vi "Shell and Tube Heat Exchanger 3.vi"() -> ()   [LabVIEW 2017]
uses:
  <vilib>/addons/control/pid/pid.llb/PID Control Input Filter (DBL).vi
  <vilib>/addons/control/pid/pid.llb/PID Advanced (DBL).vi
  <vilib>/addons/control/pid/NI_PID_pid.lvlib
panel:
  in  "stop":bool
  in  "Recording Increment (sec)":dbl=0.3 min=0.1 max=100.0 step=0.1 format="%#_13g"
  in  "error in":errorcluster
  out "Last Time Write":dbl
  in  "Replace File":bool
  out "Makeup Flowrate":dbl caption="L/min"
  out "Makeup Temperature":dbl caption="C"
  in  "Pump Switch":bool
  out "Water Outlet Temperature":dbl=22.816489944987293 format="%.1f"
  in  "Flowrate Setpoint (GPM)":dbl=40.0 min=0.0 max=50.0 format="%.2f"
  out "Water Flowrate":dbl=-0.0005338564515105265 format="%.2f"
  out "Flow Control Valve":dbl(slide)=100.0 scale=0.0..100.0
  in  "Manual Control Override (Flow)":bool=TRUE
  in  "Set Manual Valve Position (Flow)":dbl(slide)=100.0 scale=0.0..100.0
  in  "Level Setpoint (ft)":dbl=1.5 min=0.0 max=2.0 format="%.2f"
  out "Liquid Level in Tank":dbl=-0.5117058749718749 format="%.2f"
  out "Level Control Valve":dbl(slide)=0.045055175643920364 scale=0.0..100.0
  in  "Manual Control Override (Level)":bool=TRUE
  in  "Set Manual Valve Position (Level)":dbl(slide) scale=0.0..100.0
  in  "Kc (Flow)":dbl=0.74
  in  "Ti (Flow)":dbl=0.036 caption="(min)"
  in  "Td (Flow)":dbl caption="(min)"
  in  "Kc (Level)":dbl=-75.0
  in  "Ti (Level)":dbl=0.005 caption="(min)"
  in  "Td (Level)":dbl caption="(min)"
  out "House Steam Pressure":dbl=-37.74410859375 caption="psig" format="%#.6g"
  out "Tube-Side Pressure Drop":dbl=-3.6907662628125 caption="psig"
  in  "Main Power":bool
  out "Water Feed Temperature":dbl=19.10777415276108 caption="C"
  in  "Steam Pressure Setpoint (psig)":dbl=10.0 min=0.0 max=45.0 format="%.2f"
  out "Steam Pressure":dbl=-38.330115825 caption="psig" format="%.2f"
  out "Steam Valve":dbl(slide) scale=0.0..100.0
  in  "Manual Control Override (Steam Pressure)":bool
  in  "Set Manual Valve Position (Steam Pressure)":dbl(slide) scale=0.0..100.0
  in  "Kc (Steam)":dbl=0.5
  in  "Ti (Steam)":dbl=0.05 caption="(min)"
  in  "Td (Steam)":dbl caption="(min)"
  in  "Enable 5":bool
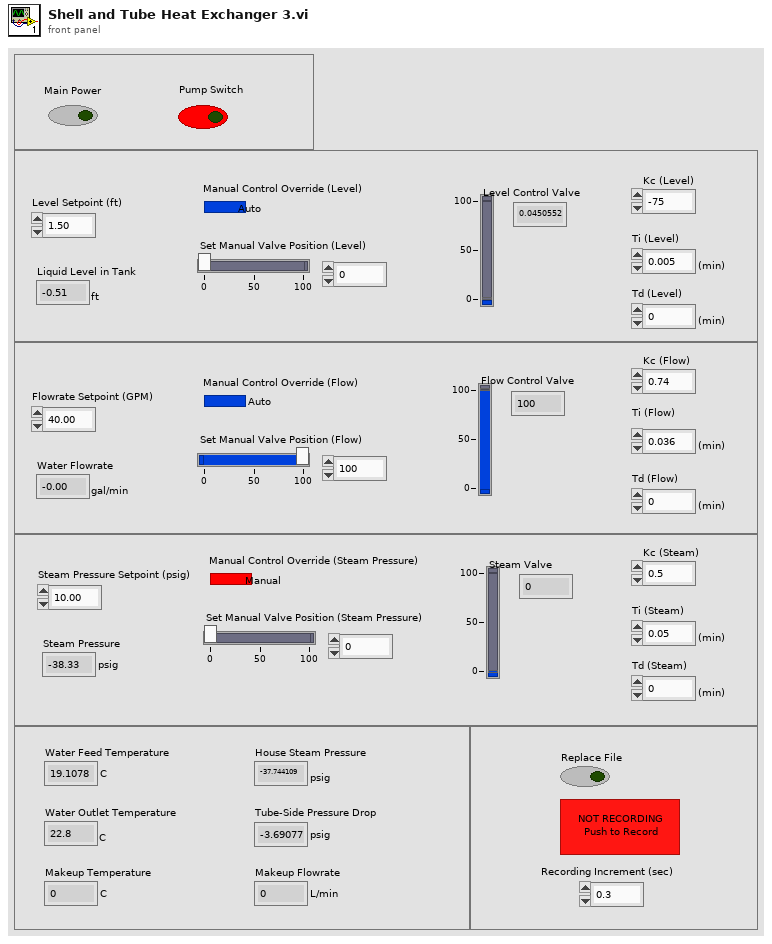
[diagram p1: front panel]
types:
  T1 = enum16{"open", "replace", "create", "open or create", "replace or create", "replace or create with confirmation"}
  T2 = cluster{"Kc (Flow)":dbl, "Ti (Flow)":dbl, "Td (Flow)":dbl}
  T3 = cluster{"Kc (Steam)":dbl, "Ti (Steam)":dbl, "Td (Steam)":dbl}
  T4 = cluster{"Kc (Level)":dbl, "Ti (Level)":dbl, "Td (Level)":dbl}
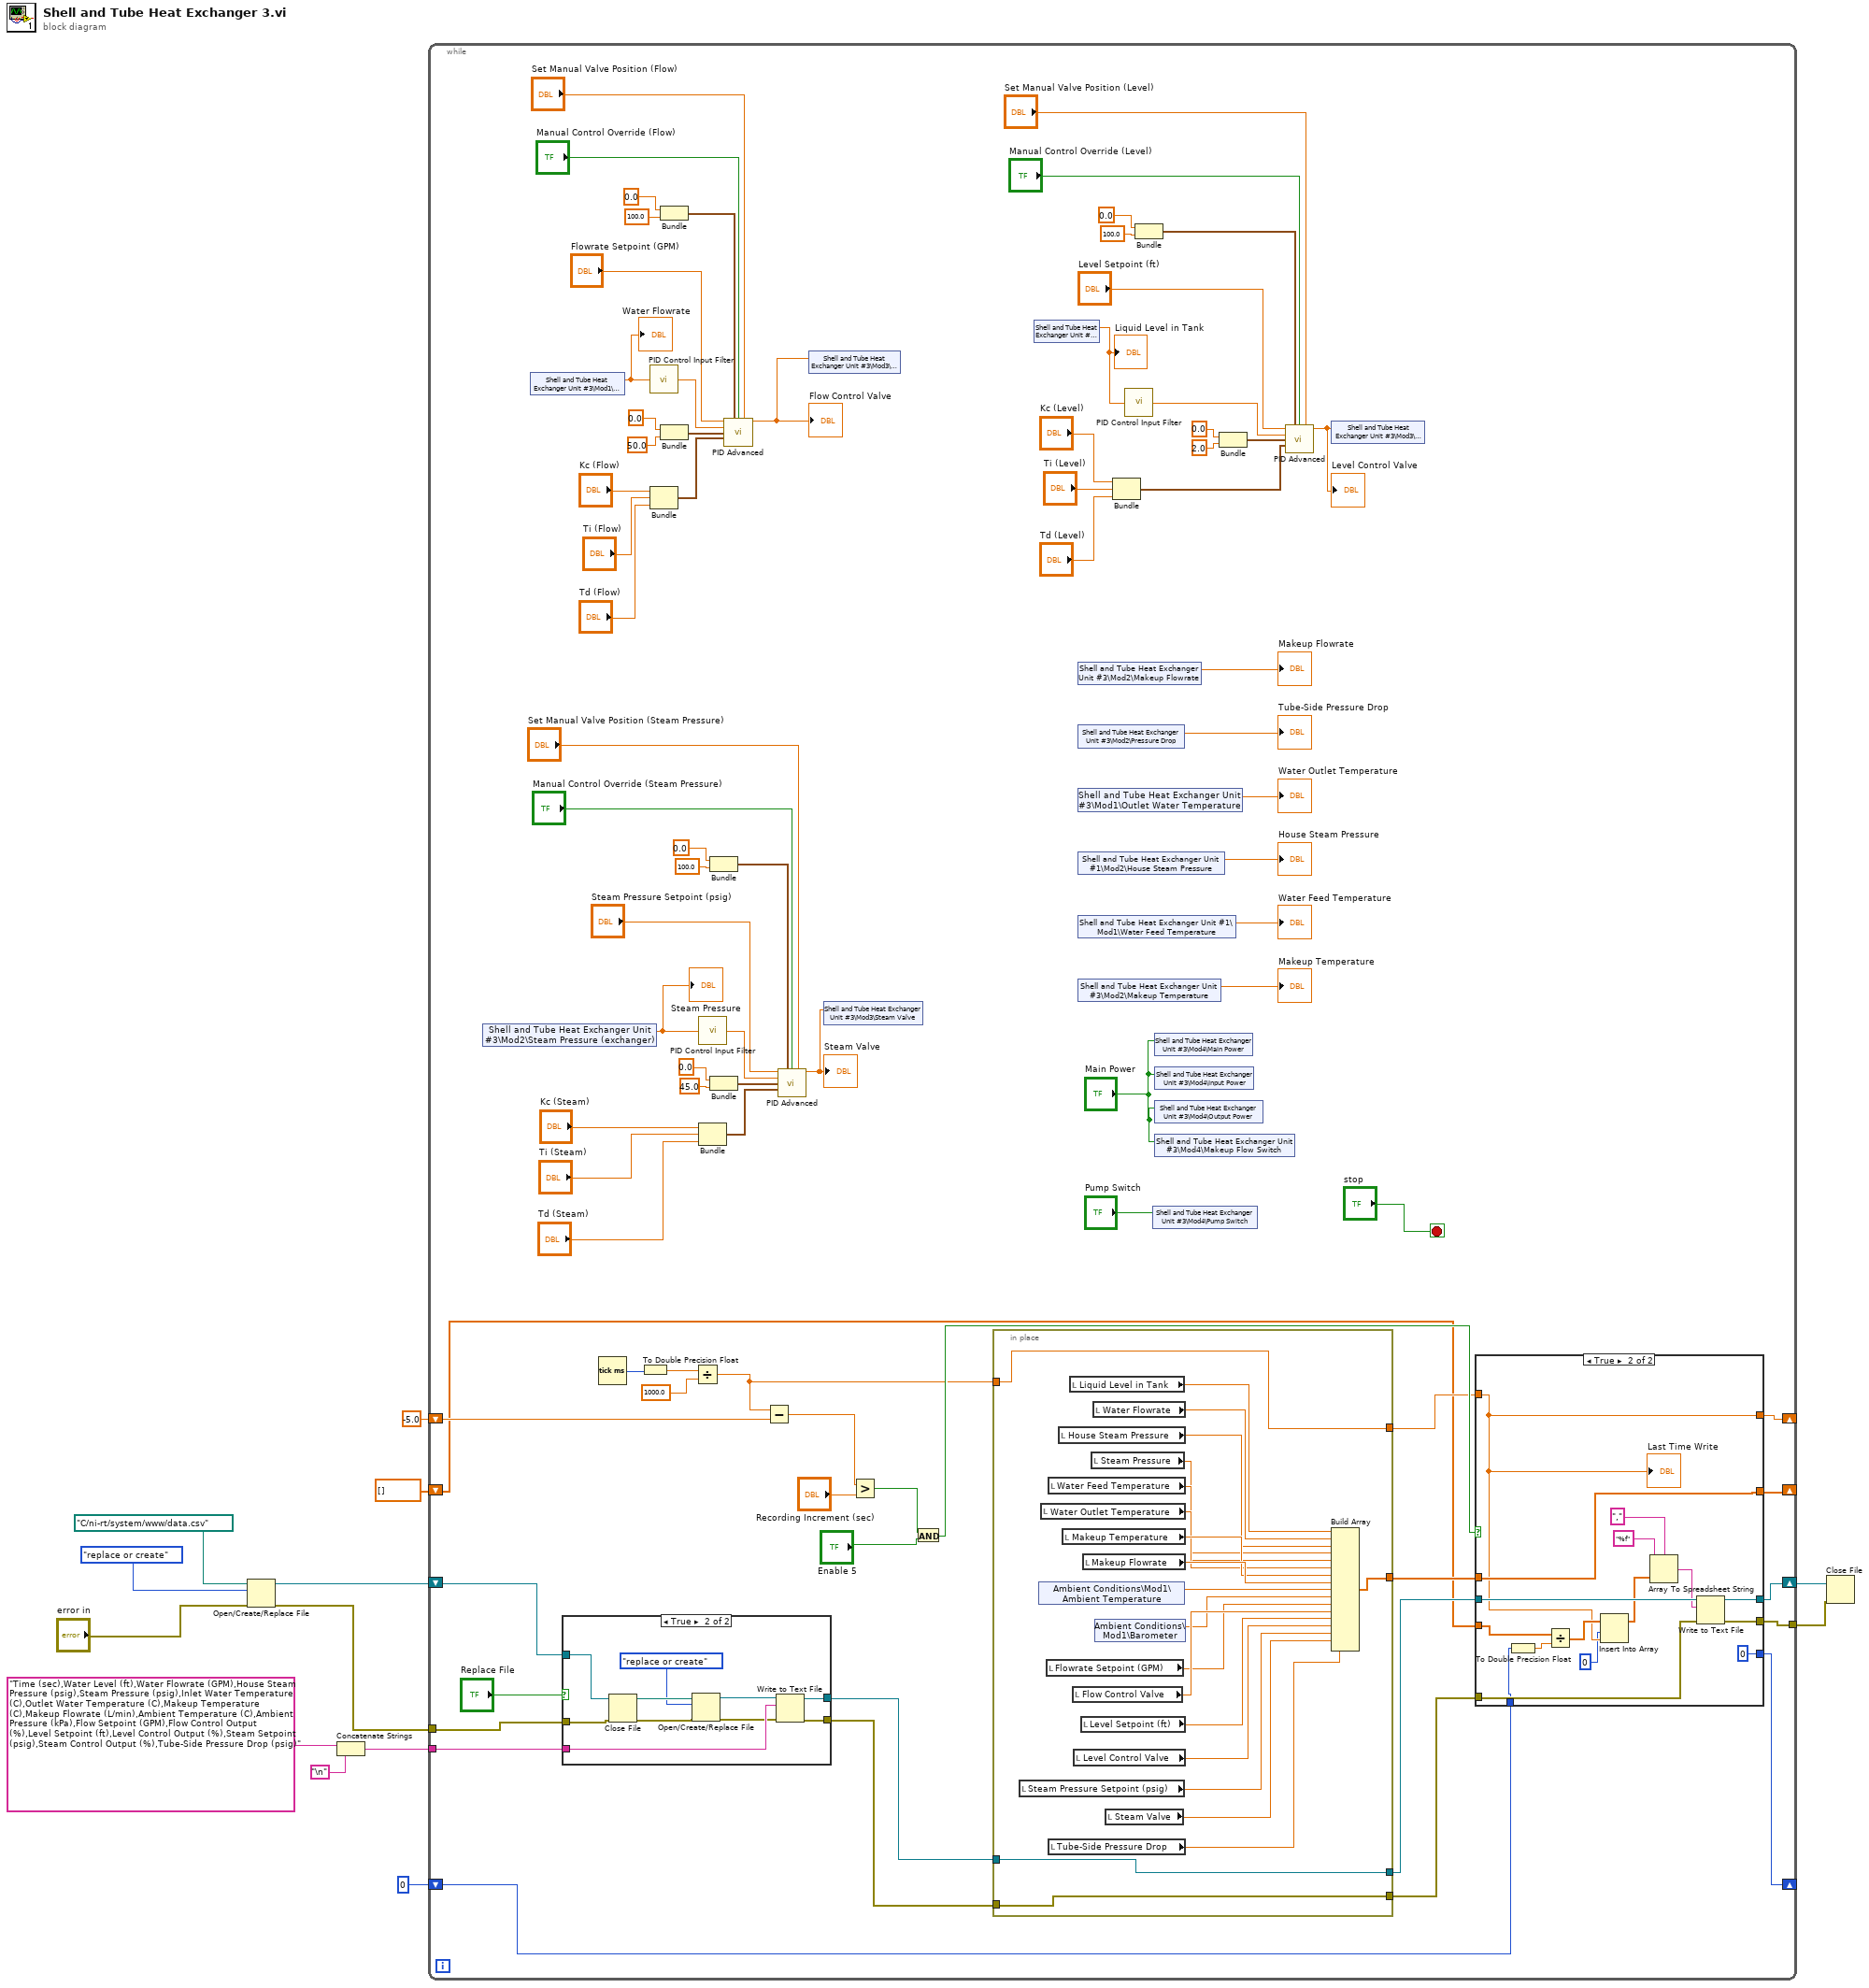
[diagram p0: block diagram]
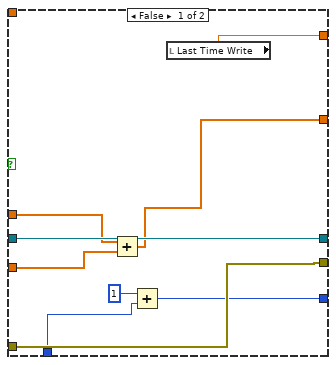
[diagram p2: hidden frame]
diagram:
  n1 = Open/Create/Replace File(file path (use dialog)=path "C:/ni-rt/system/www/data.csv" ("Filename"), error in="error in", operation (0:open)=T1."replace or create") -> (refnum out=w10:refnum<file>, error out=w5:errorcluster)  [unwired: 3 in, 1 out]
  n2 = Concatenate Strings("Time (sec),Water Level (ft),Water Flowrate (GPM),House Steam Pressure (psig),Steam Pressure (psig),Inlet Water Temperature (C),Outlet Water Temperature (C),Makeup Temperature (C),Makeup Flowrate (L/min),Ambient Temperature (C),Ambient Pressure (kPa),Flow Setpoint (GPM),Flow Control Output (%),Level Setpoint (ft),Level Control Output (%),Steam Setpoint (psig),Steam Control Output (%),Tube-Side Pressure Drop (psig)", "\n") -> (w8:string)
  n3 = while {
    tunnel: w8 -> [w41]
    shift-right: [w31] -> _
    shift-left: -5.0 ("Last Time Write") -> [w34]
    shift-right: [w29] -> w7
    shift-left: w10 -> [w40]
    tunnel: w5 -> [w28]
    tunnel: [w27] -> w4
    shift-right: [w17] -> _
    shift-left: dbl[] [] -> [w16]
    shift-right: [w14] -> _
    shift-left: 0 -> [w15]
    stop <- "stop" stop-if-true
    n4 = shared-variable "Shell and Tube Heat Exchanger Unit #3\\Mod2\\Steam Pressure (exchanger)"() -> (w52:dbl)  [unwired: 1 in, 1 out]
    "Steam Pressure" <- w52
    n5 = shared-variable "Shell and Tube Heat Exchanger Unit #3\\Mod1\\Water Flow"() -> (w54:dbl)  [unwired: 1 in, 1 out]
    "Water Flowrate" <- w54
    n6 = case shown="True" "Replace File" {
      tunnel: w41 -> [_ w153]
      tunnel: w40 -> [w145 w151]
      tunnel: [w145 w150] -> w21
      tunnel: w28 -> [w144 w149]
      tunnel: [w144 w146] -> w23
      frame False {
      }
      frame True {
        n7 = Close File(refnum=w151, error in=w149) -> (path=w154:path, error out=w148:errorcluster)
        n8 = Open/Create/Replace File(file path (use dialog)=w154, error in=w148, operation (0:open)=T1."replace or create") -> (refnum out=w155:refnum<file>, error out=w147:errorcluster)  [unwired: 3 in, 1 out]
        n9 = Write to Text File(file (use dialog)=w155, text=w153, error in=w147) -> (refnum out=w150:refnum<file>, error out=w146:errorcluster)  [unwired: 1 in, 1 out]
      }
    }
    n10 = Tick Count (ms)() -> (millisecond timer value=w33:u32)
    n11 = To Double Precision Float(number=w33) -> (double precision float=w32:dbl)
    n12 = call-poly <vilib>:"PID Control Input Filter.vi"("input"=w54) -> ("output"=w53:dbl)  [unwired: 4 in]
    n13 = Bundle("Kc (Flow)"="Kc (Flow)", "Ti (Flow)"="Ti (Flow)", "Td (Flow)"="Td (Flow)") -> (w93:T2)  [unwired: 1 in]
    n14 = Bundle(0.0, 100.0) -> (w78:cluster{dbl, dbl})  [unwired: 1 in]
    n15 = Bundle(0.0, 50.0) -> (w75:cluster{dbl, dbl})  [unwired: 1 in]
    n16 = Divide(x=w32, y=1000.0) -> (x/y=w19:dbl)
    n17 = call-poly <vilib>:"PID Control Input Filter.vi"("input"=w52) -> ("output"=w51:dbl)  [unwired: 4 in]
    n18 = Bundle("Kc (Steam)"="Kc (Steam)", "Ti (Steam)"="Ti (Steam)", "Td (Steam)"="Td (Steam)") -> (w67:T3)  [unwired: 1 in]
    n19 = Bundle(0.0, 100.0) -> (w62:cluster{dbl, dbl})  [unwired: 1 in]
    n20 = Bundle(0.0, 45.0) -> (w59:cluster{dbl, dbl})  [unwired: 1 in]
    n21 = call-poly <vilib>:"PID Advanced.vi"("setpoint"="Flowrate Setpoint (GPM)", "output range"=w78, "auto? (T)"="Manual Control Override (Flow)", "manual control"="Set Manual Valve Position (Flow)", "process variable"=w53, "setpoint range"=w75, "PID gains"=w93) -> ("output"=w49:dbl)  [unwired: 7 in, 1 out]
    "Flow Control Valve" <- w49
    n22 = Subtract(x=w19, y=w34) -> (x-y=w35:dbl)
    n23 = call-poly <vilib>:"PID Advanced.vi"("setpoint"="Steam Pressure Setpoint (psig)", "output range"=w62, "auto? (T)"="Manual Control Override (Steam Pressure)", "manual control"="Set Manual Valve Position (Steam Pressure)", "process variable"=w51, "setpoint range"=w59, "PID gains"=w67) -> ("output"=w46:dbl)  [unwired: 7 in, 1 out]
    "Steam Valve" <- w46
    n24 = shared-variable "Shell and Tube Heat Exchanger Unit #3\\Mod3\\Flow Valve"(w49) -> ()  [unwired: 1 in, 1 out]
    n25 = shared-variable "Shell and Tube Heat Exchanger Unit #3\\Mod3\\Steam Valve"(w46) -> ()  [unwired: 1 in, 1 out]
    n26 = Greater?(x=w35, y="Recording Increment (sec)") -> (0:w37:bool)
    n27 = And(x=w37, y="Enable 5") -> (x .and. y?=w38:bool)
    n28 = in-place {
      in-place-border: [w101] -> w24
      in-place-border: w23 -> [w101]
      in-place-border: [w100] -> w22
      in-place-border: w21 -> [w100]
      in-place-border: [w99] -> w20
      in-place-border: w19 -> [w98]
      in-place-border: [w98] -> w18
      n29 = local read "Steam Pressure Setpoint (psig)"() -> (w116:dbl)
      n30 = shared-variable "Ambient Conditions\\Mod1\\Ambient Temperature"() -> (w110:dbl)  [unwired: 1 in, 1 out]
      n31 = local read "Water Outlet Temperature"() -> (w107:dbl)
      n32 = local read "Flowrate Setpoint (GPM)"() -> (w112:dbl)
      n33 = local read "Water Feed Temperature"() -> (w106:dbl)
      n34 = local read "Tube-Side Pressure Drop"() -> (w118:dbl)
      n35 = local read "House Steam Pressure"() -> (w104:dbl)
      n36 = local read "Makeup Temperature"() -> (w108:dbl)
      n37 = local read "Liquid Level in Tank"() -> (w102:dbl)
      n38 = local read "Flow Control Valve"() -> (w113:dbl)
      n39 = local read "Level Control Valve"() -> (w115:dbl)
      n40 = local read "Level Setpoint (ft)"() -> (w114:dbl)
      n41 = local read "Makeup Flowrate"() -> (w109:dbl)
      n42 = local read "Steam Pressure"() -> (w105:dbl)
      n43 = local read "Water Flowrate"() -> (w103:dbl)
      n44 = shared-variable "Ambient Conditions\\Mod1\\Barometer"() -> (w111:dbl)  [unwired: 1 in, 1 out]
      n45 = local read "Steam Valve"() -> (w117:dbl)
      n46 = Build Array(w102, w103, w104, w105, w106, w107, w108, w109, w110, w111, w112, w113, w114, w115, w116, w117, w118) -> (w99:dbl[])
    }
    n47 = shared-variable "Shell and Tube Heat Exchanger Unit #3\\Mod2\\Level"() -> (w56:dbl)  [unwired: 1 in, 1 out]
    "Liquid Level in Tank" <- w56
    n48 = shared-variable "Shell and Tube Heat Exchanger Unit #3\\Mod2\\Makeup Flowrate"() -> (→"Makeup Flowrate":dbl)  [unwired: 1 in, 1 out]
    n49 = shared-variable "Shell and Tube Heat Exchanger Unit #3\\Mod2\\Pressure Drop"() -> (→"Tube-Side Pressure Drop":dbl)  [unwired: 1 in, 1 out]
    n50 = shared-variable "Shell and Tube Heat Exchanger Unit #3\\Mod1\\Outlet Water Temperature"() -> (→"Water Outlet Temperature":dbl)  [unwired: 1 in, 1 out]
    n51 = shared-variable "Shell and Tube Heat Exchanger Unit #1\\Mod2\\House Steam Pressure"() -> (→"House Steam Pressure":dbl)  [unwired: 1 in, 1 out]
    n52 = shared-variable "Shell and Tube Heat Exchanger Unit #1\\Mod1\\Water Feed Temperature"() -> (→"Water Feed Temperature":dbl)  [unwired: 1 in, 1 out]
    n53 = shared-variable "Shell and Tube Heat Exchanger Unit #3\\Mod2\\Makeup Temperature"() -> (→"Makeup Temperature":dbl)  [unwired: 1 in, 1 out]
    n54 = Bundle("Kc (Level)"="Kc (Level)", "Ti (Level)"="Ti (Level)", "Td (Level)"="Td (Level)") -> (w95:T4)  [unwired: 1 in]
    n55 = call-poly <vilib>:"PID Control Input Filter.vi"("input"=w56) -> ("output"=w55:dbl)  [unwired: 4 in]
    n56 = Bundle(0.0, 100.0) -> (w81:cluster{dbl, dbl})  [unwired: 1 in]
    n57 = shared-variable "Shell and Tube Heat Exchanger Unit #3\\Mod4\\Pump Switch"("Pump Switch") -> ()  [unwired: 1 in, 1 out]
    n58 = shared-variable "Shell and Tube Heat Exchanger Unit #3\\Mod4\\Main Power"("Main Power") -> ()  [unwired: 1 in, 1 out]
    n59 = shared-variable "Shell and Tube Heat Exchanger Unit #3\\Mod4\\Input Power"("Main Power") -> ()  [unwired: 1 in, 1 out]
    n60 = shared-variable "Shell and Tube Heat Exchanger Unit #3\\Mod4\\Output Power"("Main Power") -> ()  [unwired: 1 in, 1 out]
    n61 = shared-variable "Shell and Tube Heat Exchanger Unit #3\\Mod4\\Makeup Flow Switch"("Main Power") -> ()  [unwired: 1 in, 1 out]
    n62 = Bundle(0.0, 2.0) -> (w72:cluster{dbl, dbl})  [unwired: 1 in]
    n63 = call-poly <vilib>:"PID Advanced.vi"("setpoint"="Level Setpoint (ft)", "output range"=w81, "auto? (T)"="Manual Control Override (Level)", "manual control"="Set Manual Valve Position (Level)", "process variable"=w55, "setpoint range"=w72, "PID gains"=w95) -> ("output"=w48:dbl)  [unwired: 7 in, 1 out]
    "Level Control Valve" <- w48
    n64 = shared-variable "Shell and Tube Heat Exchanger Unit #3\\Mod3\\Level Valve"(w48) -> ()  [unwired: 1 in, 1 out]
    n65 = case shown="True" w38 {
      tunnel: w22 -> [w126 w140]
      tunnel: [w126 w143] -> w29
      tunnel: w18 -> [_ w130]
      tunnel: [w127 w130] -> w31
      tunnel: w24 -> [w125 w142]
      tunnel: [w125 w141] -> w27
      tunnel: w20 -> [w124 w132]
      tunnel: [w122 w132] -> w17
      tunnel: w16 -> [w123 w134]
      tunnel: w15 -> [w121 w135]
      tunnel: [w119 0] -> w14
      frame False {
        n66 = Add(x=w124, y=w123) -> (x+y=w122:dbl[])
        n67 = Add(x=1, y=w121) -> (x+y=w119:i32)
        n68 = local read "Last Time Write"() -> (w127:dbl)
      }
      frame True {
        n69 = To Double Precision Float(number=w135) -> (double precision float=w136:dbl)
        n70 = Divide(x=w134, y=w136) -> (x/y=w131:dbl[])
        n71 = Insert Into Array(array=w131, index=0, new element=w130) -> (w129:dbl[])
        n72 = Array To Spreadsheet String(delimiter (Tab)=",", array=w129, 3:"%f") -> (spreadsheet string=w137:string)
        n73 = Write to Text File(file (use dialog)=w140, text=w137, error in=w142) -> (refnum out=w143:refnum<file>, error out=w141:errorcluster)  [unwired: 1 in, 1 out]
        "Last Time Write" <- w130
      }
    }
  }
  n74 = Close File(refnum=w7, error in=w4) -> ()  [unwired: 2 out]
